vi "Phasor Get Phasor Ratio.vi"(6 "Phasor SDV":T1={"g"=nan, "s"=nan}, 7 "z":cdb=nan+nani, 8 "Error In":errorcluster, 9 "Reference Phasor 2":T1, 10 "Reference Phasor 1":T1, 11 "Phasor":T1={"g"=nan, "s"=nan}) -> (0 "Error Out":errorcluster, 1 "Phasor Ratio SDV":dbl, 3 "Phasor Ratio (f1)":dbl)   [LabVIEW 2021, in "Phasor.lvlib"]
doc: "Computes the phasor ratio based on phasor references 1 and 2.\nIf <B>z</B> is not connected, the <B>Phasor</B> cluster is used instead."
uses:
  Phasor.lvlib
  Phasor (g, s).ctl
panel:
  # "see the License on the block diagram (Ctrl+E or Window:Show Block Diagram)"
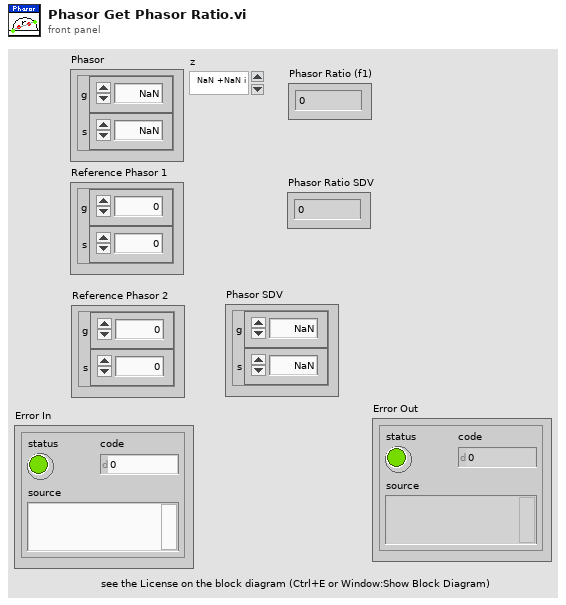
[diagram p1: front panel]
types:
  T1 = typedef "Phasor.lvlib/Phasor (g, s).ctl" = cluster{"g":dbl, "s":dbl}
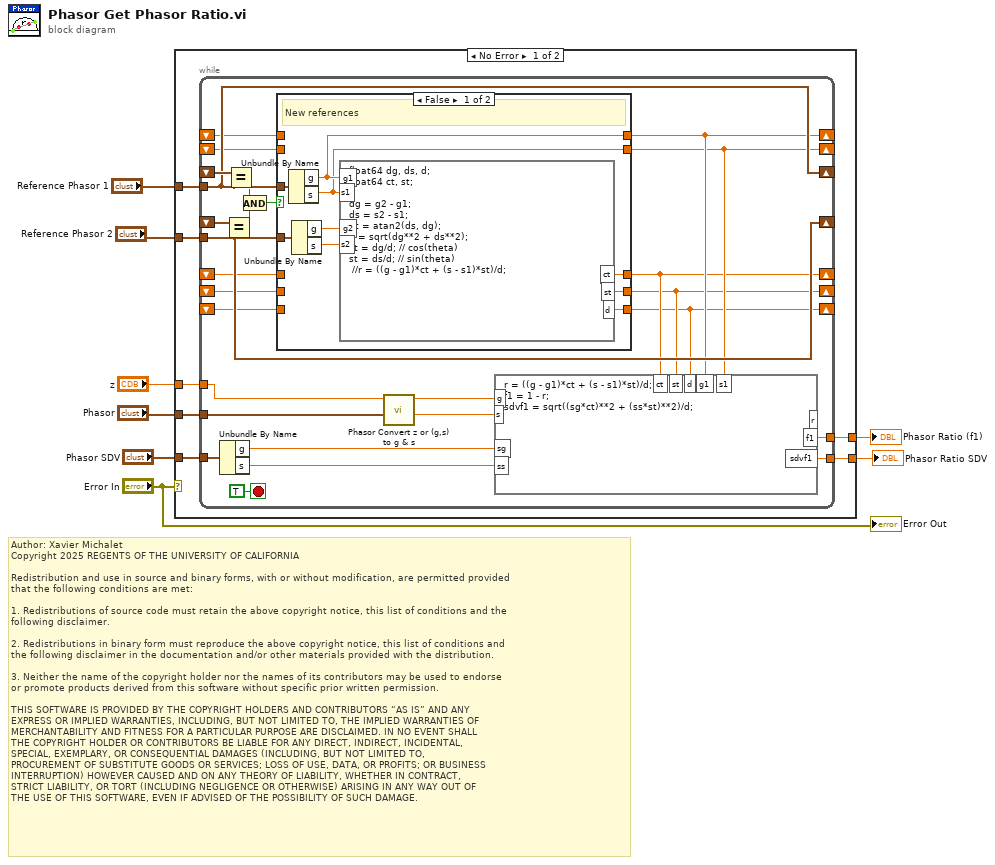
[diagram p0: block diagram]
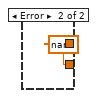
[diagram p3: hidden frame]
diagram:
  # "Author: Xavier Michalet\nCopyright 2025 REGENTS OF THE UNIVERSITY OF CALIFORNIA\n\nRedistribution and use in source and binary forms, with or without modification, are permitted provided\nthat the following conditions are met:\n\n1. Redistributions of source code must retain the above copyright notice, this list of conditions and the\nfollowing disclaimer.\n\n2. Redistributions in binary form must reproduce the above copyright notice, this list of conditions and\nthe following disclaimer in the documentation and/or other materials provided with the distribution.\n\n3. Neither the name of the copyright holder nor the names of its contributors may be used to endorse \nor promote products derived from this software without specific prior written permission.\n\nTHIS SOFTWARE IS PROVIDED BY THE COPYRIGHT HOLDERS AND CONTRIBUTORS “AS IS” AND ANY \nEXPRESS OR IMPLIED WARRANTIES, INCLUDING, BUT NOT LIMITED TO, THE IMPLIED WARRANTIES OF\nMERCHANTABILITY AND FITNESS FOR A PARTICULAR PURPOSE ARE DISCLAIMED. IN NO EVENT SHALL\nTHE COPYRIGHT HOLDER OR CONTRIBUTORS BE LIABLE FOR ANY DIRECT, INDIRECT, INCIDENTAL, \nSPECIAL, EXEMPLARY, OR CONSEQUENTIAL DAMAGES (INCLUDING, BUT NOT LIMITED TO, \nPROCUREMENT OF SUBSTITUTE GOODS OR SERVICES; LOSS OF USE, DATA, OR PROFITS; OR BUSINESS\nINTERRUPTION) HOWEVER CAUSED AND ON ANY THEORY OF LIABILITY, WHETHER IN CONTRACT, \nSTRICT LIABILITY, OR TORT (INCLUDING NEGLIGENCE OR OTHERWISE) ARISING IN ANY WAY OUT OF\nTHE USE OF THIS SOFTWARE, EVEN IF ADVISED OF THE POSSIBILITY OF SUCH DAMAGE."
  n1 = case shown="No Error" "Error In" {
    tunnel: "Reference Phasor 2" -> [w15 _]
    tunnel: "Reference Phasor 1" -> [w14 _]
    tunnel: "Phasor" -> [w13 _]
    tunnel: [w12 w57] -> w5
    tunnel: "z" -> [w11 _]
    tunnel: "Phasor SDV" -> [w10 _]
    tunnel: [w9 w57] -> w1
    frame No Error {
      n2 = while {
        tunnel: w15 -> [w40]
        tunnel: w14 -> [w38]
        tunnel: w13 -> [w17]
        shift-right: [w38] -> _
        shift-left: _ -> [w39]
        shift-right: [w40] -> _
        shift-left: _ -> [w41]
        shift-right: [w27] -> _
        shift-left: _ -> [w34]
        shift-right: [w26] -> _
        shift-left: _ -> [w33]
        shift-right: [w25] -> _
        shift-left: _ -> [w32]
        shift-right: [w29] -> _
        shift-left: _ -> [w31]
        shift-right: [w28] -> _
        shift-left: _ -> [w30]
        tunnel: [w23] -> w12
        tunnel: w11 -> [w22]
        tunnel: w10 -> [w21]
        tunnel: [w18] -> w9
        stop <- TRUE stop-if-true
        n3 = Unbundle By Name(w21) -> ("g"=w20:dbl, "s"=w19:dbl)
        n4 = Equal?(x=w41, y=w40) -> (x = y?=w37:bool)
        n5 = Equal?(x=w39, y=w38) -> (x = y?=w36:bool)
        n6 = And(x=w36, y=w37) -> (x .and. y?=w35:bool)
        n7 = case shown="False" w35 {
          tunnel: w40 -> [w51 _]
          tunnel: w38 -> [w50 _]
          tunnel: [w47 w54] -> w25
          tunnel: [w46 w55] -> w26
          tunnel: [w45 w56] -> w27
          tunnel: w34 -> [_ w56]
          tunnel: w33 -> [_ w55]
          tunnel: w32 -> [_ w54]
          tunnel: [w44 w53] -> w29
          tunnel: [w43 w52] -> w28
          tunnel: w31 -> [_ w53]
          tunnel: w30 -> [_ w52]
          frame False {
            # "New references"
            n8 = Unbundle By Name(w50) -> ("g"=w44:dbl, "s"=w43:dbl)
            n9 = Unbundle By Name(w51) -> ("g"=w49:dbl, "s"=w48:dbl)
            n10 = formula code="float64 dg, ds, d;\nfloat64 ct, st;\n\ndg = g2 - g1;\nds = s2 - s1;\n//t = atan2(ds, dg);\nd = sqrt(dg**2 + ds**2);\nct = dg/d; // cos(theta)\nst = ds/d; // sin(theta)\n //r = ((g - g1)*ct + (s - s1)*st)/d;"("g1"=w44, "s1"=w43, "g2"=w49, "s2"=w48) -> ("ct"=w45:dbl, "st"=w46:dbl, "d"=w47:dbl)
          }
          frame True {
            # "same references"
          }
        }
        n11 = call "Phasor Convert z or (g,s) to g & s.vi"("Phasor"=w17, "z"=w22) -> ("s"=w16:dbl, "g"=w24:dbl)  [unwired: 8 in]
        n12 = formula code="r = ((g - g1)*ct + (s - s1)*st)/d;\nf1 = 1 - r;\nsdvf1 = sqrt((sg*ct)**2 + (ss*st)**2)/d;"("g1"=w29, "s1"=w28, "g"=w24, "s"=w16, "ct"=w27, "st"=w26, "d"=w25, "sg"=w20, "ss"=w19) -> ("f1"=w23:dbl, "sdvf1"=w18:dbl)  [unwired: 1 out]
      }
    }
    frame Error {
      w57 = nan ("r")
    }
  }
  "Phasor Ratio (f1)" <- w5
  "Phasor Ratio SDV" <- w1
  "Error Out" <- "Error In"
